vi "LEDBlinker.vi"(8 "Timings":sgl[](array[numeric]), 10 "Color 2":u32, 11 "Color 1":u32) -> (3 "Color out":u32)   [LabVIEW 2020]
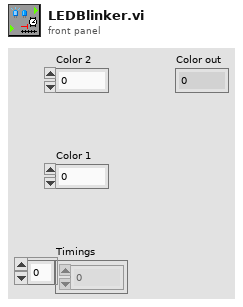
[diagram p1: front panel]
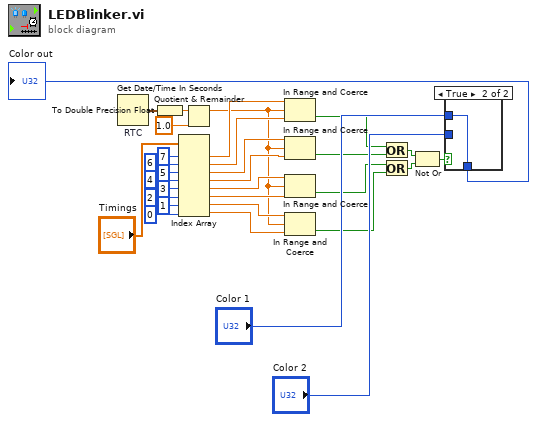
[diagram p0: block diagram]
diagram:
  n1 = Get Date/Time In Seconds "RTC"() -> (seconds since 1Jan1904=w31:timestamp)
  n2 = To Double Precision Float(number=w31) -> (double precision float=w2:dbl)
  n3 = Index Array(array="Timings", index #1=7 ("index"), index #2=6 ("index"), index #3=5 ("index"), index #4=4 ("index"), index #5=3 ("index"), index #6=2 ("index"), index #7=1 ("index"), index #8=0 ("index")) -> (element #1=w21:sgl, element #2=w20:sgl, element #3=w19:sgl, element #4=w18:sgl, element #5=w17:sgl, element #6=w16:sgl, element #7=w15:sgl, element #8=w14:sgl)
  n4 = Quotient & Remainder(x=w2, y=1.0) -> (x-y*floor(x/y)=w13:dbl)  [unwired: 1 out]
  n5 = In Range and Coerce(upper limit=w21, x=w13, lower limit=w20) -> (In Range?=w25:bool)  [unwired: 1 out]
  n6 = In Range and Coerce(upper limit=w19, x=w13, lower limit=w18) -> (In Range?=w26:bool)  [unwired: 1 out]
  n7 = In Range and Coerce(upper limit=w17, x=w13, lower limit=w16) -> (In Range?=w27:bool)  [unwired: 1 out]
  n8 = In Range and Coerce(upper limit=w15, x=w13, lower limit=w14) -> (In Range?=w28:bool)  [unwired: 1 out]
  n9 = Or(x=w25, y=w26) -> (x .or. y?=w23:bool)
  n10 = Or(x=w27, y=w28) -> (x .or. y?=w24:bool)
  n11 = Not Or(1:w24, 2:w23) -> (0:w22:bool)
  n12 = case shown="True" w22 {
    tunnel: [w32 w33] -> w1
    tunnel: "Color 2" -> [w32 _]
    tunnel: "Color 1" -> [_ w33]
    frame False {
    }
    frame True {
    }
  }
  "Color out" <- w1
